vi "construct data interface.vi"(8 "error in":errorcluster, 10 "allocation specification":T1[](array[typedef])) -> (0 "error out":errorcluster, 3 "data table out":T3)   [LabVIEW 2013, in "tag bus.lvlib" / "data table.lvlib"]
doc: "Creates a data table based on the number of tags provided by the allocation specification."
uses:
  data table.lvlib
  data table.ctl
  allocation specification.ctl
  tag/Data Type.ctl
  tag/tag descriptor.lvclass
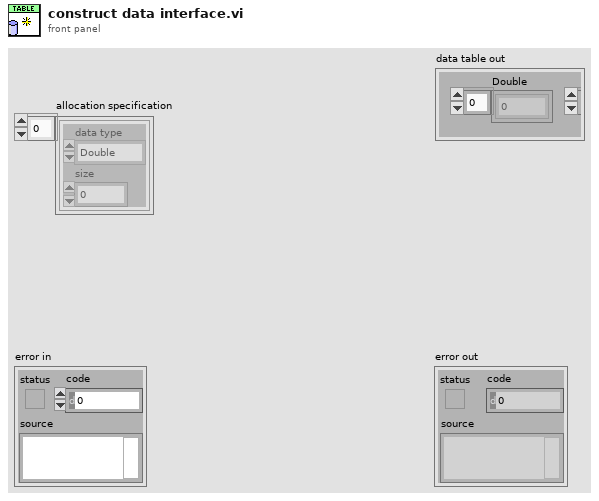
[diagram p1: front panel]
types:
  T1 = typedef "tag bus.lvlib/data table.lvlib/allocation specification.ctl" = cluster{"data type":T2, "size":i32}
  T2 = typedef "tag bus.lvlib/tag descriptor.lvclass/Data Type.ctl" = enum16{"Double", "Single", "I64", "I32", "I16", "I8", "U64", "U32", "U16", "U8", "Boolean", "String", "Array of Double", "Array of Single", "Array of I64", "Array of I32", "Array of I16", "Array of I8", "Array of U64", "Array of U32", "Array of U16", "Array of U8", "Array of Boolean", "Array of String"}
  T3 = typedef "tag bus.lvlib/data table.lvlib/data table.ctl" = cluster{"Double":dbl[], "Single":sgl[], "I64":i64[], "I32":i32[], "I16":i16[], "I8":i8[], "U64":u64[], "U32":u32[], "U16":u16[], "U8":u8[], "Boolean":bool[], "String":string[], "Array of Double":cluster{"DBL Array":dbl[]}[], "Array of Single":cluster{"SGL Array":sgl[]}[], "Array of I64":cluster{"I64 Array":i64[]}[], "Array of I32":cluster{"I32 Array":i32[]}[], "Array of I16":cluster{"I16 Array":i16[]}[], "Array of I8":cluster{"I8 Array":i8[]}[], "Array of U64":cluster{"U64 Array":u64[]}[], "Array of U32":cluster{"U32 Array":u32[]}[], "Array of U16":cluster{"U16 Array":u16[]}[], "Array of U8":cluster{"U8 Array":u8[]}[], "Array of Boolean":cluster{"Boolean Array":bool[]}[], "Array of String":cluster{"String Array":string[]}[]}
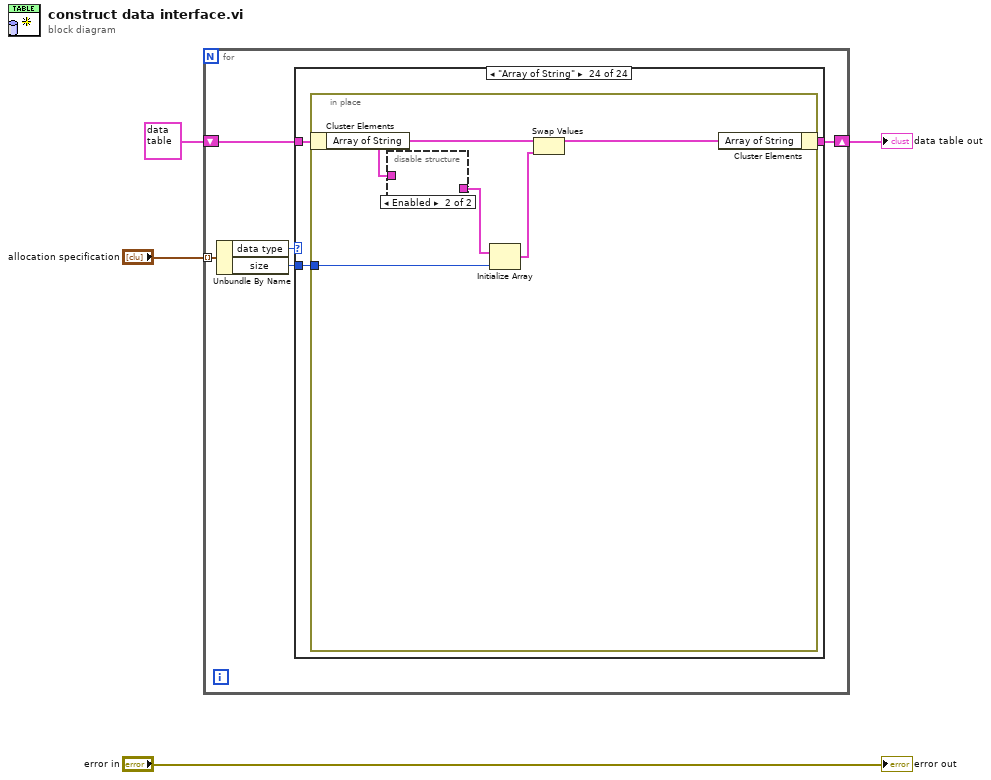
[diagram p0: block diagram]
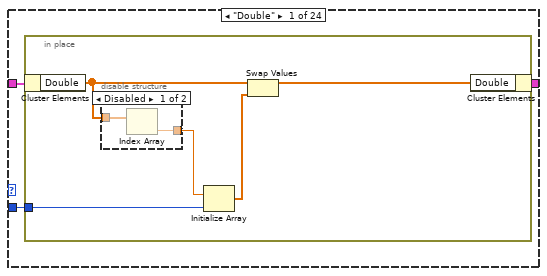
[diagram p2: hidden frame]
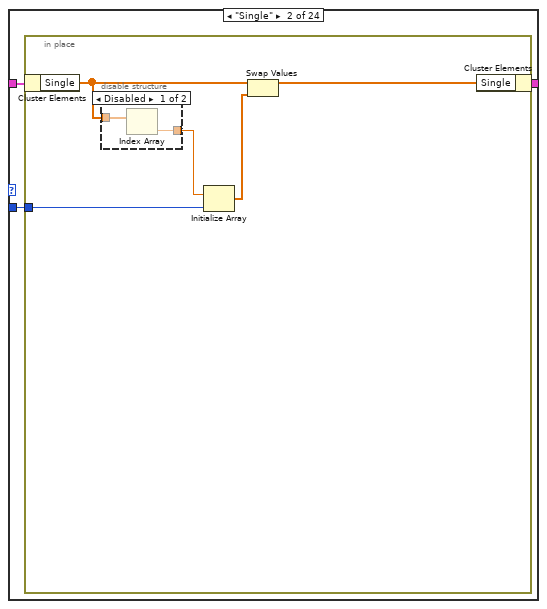
[diagram p4: hidden frame]
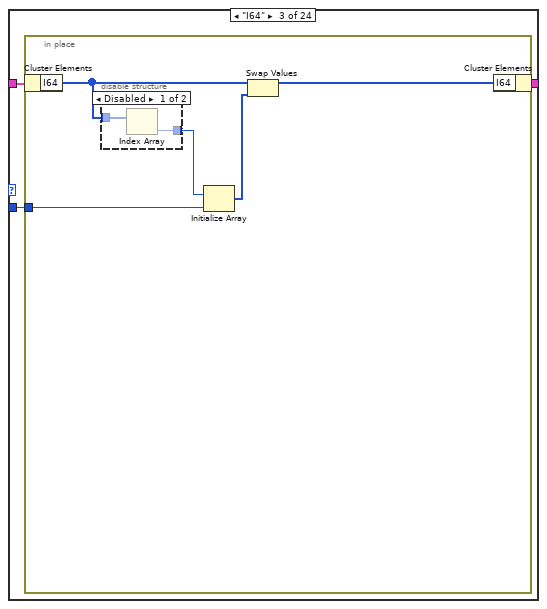
[diagram p6: hidden frame]
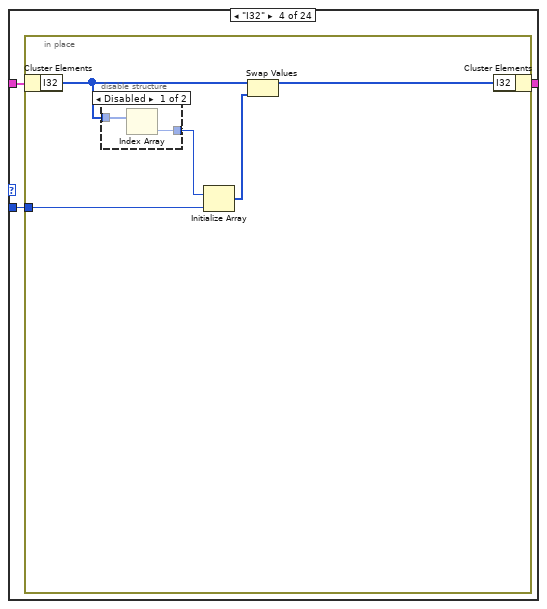
[diagram p8: hidden frame]
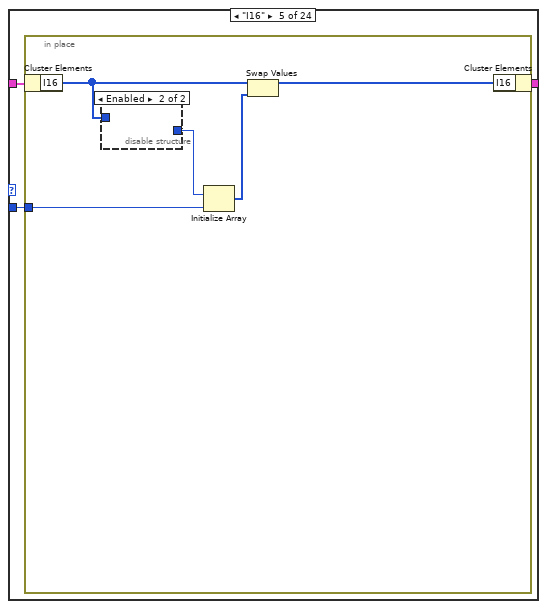
[diagram p10: hidden frame]
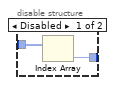
[diagram p11: hidden frame]
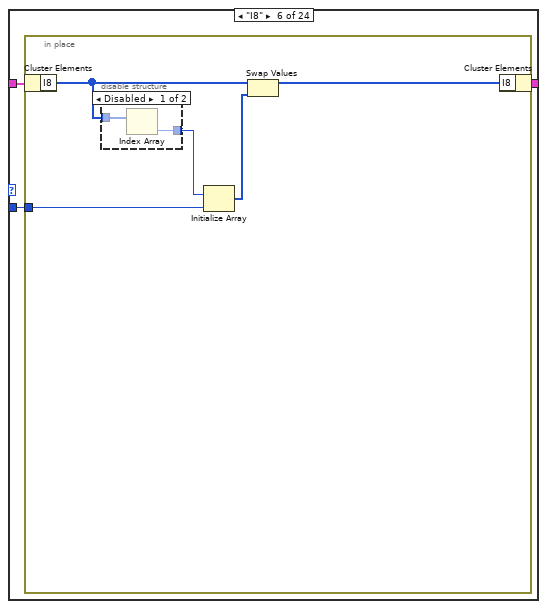
[diagram p12: hidden frame]
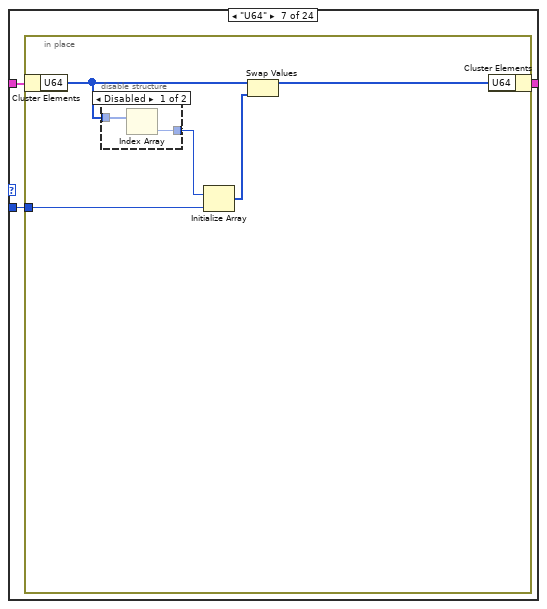
[diagram p14: hidden frame]
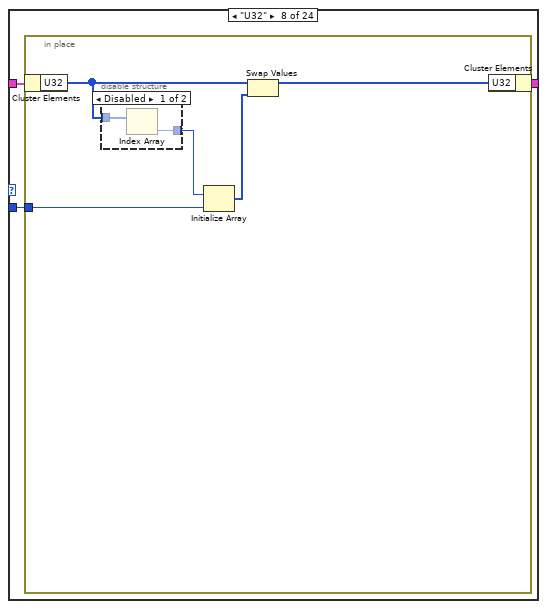
[diagram p16: hidden frame]
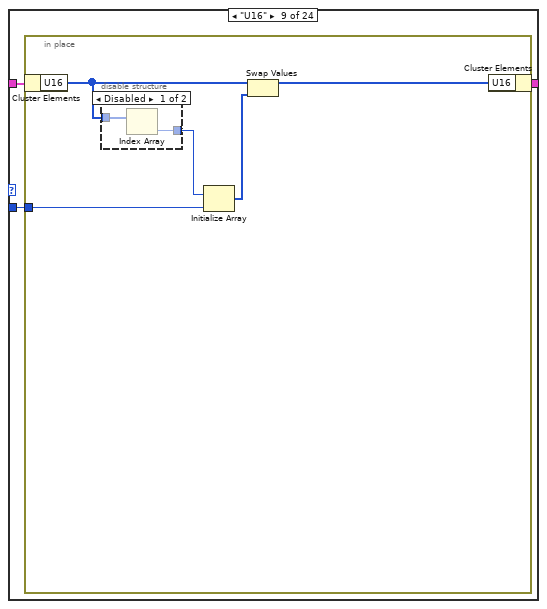
[diagram p18: hidden frame]
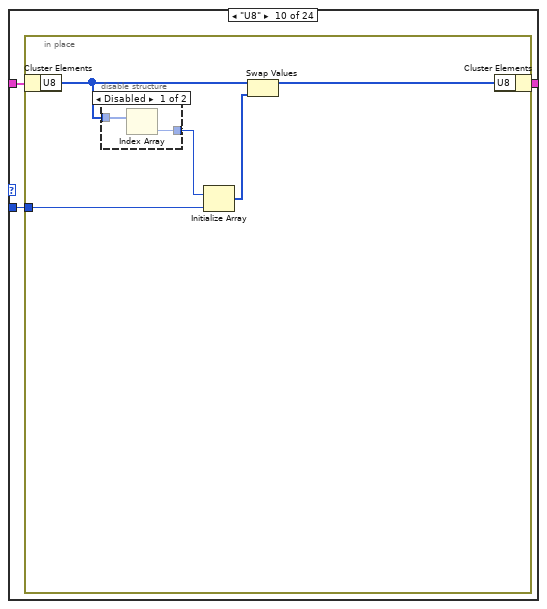
[diagram p20: hidden frame]
diagram:
  n1 = for {
    shift-right: [w6] -> w2
    shift-left: T3 {"Double"=[], "Single"=[], "I64"=[], "I32"=[], "I16"=[], "I8"=[], "U64"=[], "U32"=[], "U16"=[], "U8"=[], "Boolean"=[], "String"=[], "Array of Double"=[], "Array of Single"=[], "Array of I64"=[], "Array of I32"=[], "Array of I16"=[], "Array of I8"=[], "Array of U64"=[], "Array of U32"=[], "Array of U16"=[], "Array of U8"=[], "Array of Boolean"=[], "Array of String"=[]} ("Data Interface in") -> [w7]
    tunnel: "allocation specification" -> [w9] mode=indexing
    n2 = Unbundle By Name(w9) -> ("data type"=w8:T2, "size"=w5:i32)
    n3 = case shown="\"Array of String\"" w8 {
      tunnel: w7 -> [w11 w21 w31 w41 w51 w61 w71 w81 w91 w101 w111 w121 w131 w141 w151 w161 w171 w181 w191 w201 w211 w221 w231 w241]
      tunnel: [w12 w22 w32 w42 w52 w62 w72 w82 w92 w102 w112 w122 w132 w142 w152 w162 w172 w182 w192 w202 w212 w222 w232 w242] -> w6
      tunnel: w5 -> [w10 w20 w30 w40 w50 w60 w70 w80 w90 w100 w110 w120 w130 w140 w150 w160 w170 w180 w190 w200 w210 w220 w230 w240]
      frame "Double" {
        n4 = in-place {
          in-place-border: w10 -> [w17]
          n5 = in-place-cluster #1(w11) -> ("Double"=w15:dbl[])
          n6 = disable-structure shown="Disabled" {
            disable-tunnel: w15 -> [w19 _]
            disable-tunnel: [w18 _] -> w16
            frame Disabled {
              n7 = Index Array(array=w19) -> (element=w18:dbl)  [unwired: 1 in]
            }
            frame Enabled {
            }
          }
          n8 = Initialize Array(w16, w17) -> (w13:dbl[])
          n9 = Swap Values(12:w15, 14:w13) -> (1:w14:dbl[])  [unwired: 1 in, 1 out]
          n10 = in-place-cluster #1("Double"=w14) -> (w12:T3)
        }
      }
      frame "Single" {
        n11 = in-place {
          in-place-border: w20 -> [w27]
          n12 = in-place-cluster #2(w21) -> ("Single"=w25:sgl[])
          n13 = disable-structure shown="Disabled" {
            disable-tunnel: w25 -> [w29 _]
            disable-tunnel: [w28 _] -> w26
            frame Disabled {
              n14 = Index Array(array=w29) -> (element=w28:sgl)  [unwired: 1 in]
            }
            frame Enabled {
            }
          }
          n15 = Initialize Array(w26, w27) -> (w23:sgl[])
          n16 = Swap Values(12:w25, 14:w23) -> (1:w24:sgl[])  [unwired: 1 in, 1 out]
          n17 = in-place-cluster #2("Single"=w24) -> (w22:T3)
        }
      }
      frame "I64" {
        n18 = in-place {
          in-place-border: w30 -> [w37]
          n19 = in-place-cluster #3(w31) -> ("I64"=w35:i64[])
          n20 = disable-structure shown="Disabled" {
            disable-tunnel: w35 -> [w39 _]
            disable-tunnel: [w38 _] -> w36
            frame Disabled {
              n21 = Index Array(array=w39) -> (element=w38:i64)  [unwired: 1 in]
            }
            frame Enabled {
            }
          }
          n22 = Initialize Array(w36, w37) -> (w33:i64[])
          n23 = Swap Values(12:w35, 14:w33) -> (1:w34:i64[])  [unwired: 1 in, 1 out]
          n24 = in-place-cluster #3("I64"=w34) -> (w32:T3)
        }
      }
      frame "I32" {
        n25 = in-place {
          in-place-border: w40 -> [w47]
          n26 = in-place-cluster #4(w41) -> ("I32"=w45:i32[])
          n27 = disable-structure shown="Disabled" {
            disable-tunnel: w45 -> [w49 _]
            disable-tunnel: [w48 _] -> w46
            frame Disabled {
              n28 = Index Array(array=w49) -> (element=w48:i32)  [unwired: 1 in]
            }
            frame Enabled {
            }
          }
          n29 = Initialize Array(w46, w47) -> (w43:i32[])
          n30 = Swap Values(12:w45, 14:w43) -> (1:w44:i32[])  [unwired: 1 in, 1 out]
          n31 = in-place-cluster #4("I32"=w44) -> (w42:T3)
        }
      }
      frame "I16" {
        n32 = in-place {
          in-place-border: w50 -> [w57]
          n33 = in-place-cluster #5(w51) -> ("I16"=w55:i16[])
          n34 = disable-structure shown="Enabled" {
            disable-tunnel: w55 -> [w59 _]
            disable-tunnel: [w58 _] -> w56
            frame Disabled {
              n35 = Index Array(array=w59) -> (element=w58:i16)  [unwired: 1 in]
            }
            frame Enabled {
            }
          }
          n36 = Initialize Array(w56, w57) -> (w53:i16[])
          n37 = Swap Values(12:w55, 14:w53) -> (1:w54:i16[])  [unwired: 1 in, 1 out]
          n38 = in-place-cluster #5("I16"=w54) -> (w52:T3)
        }
      }
      frame "I8" {
        n39 = in-place {
          in-place-border: w60 -> [w67]
          n40 = in-place-cluster #6(w61) -> ("I8"=w65:i8[])
          n41 = disable-structure shown="Disabled" {
            disable-tunnel: w65 -> [w69 _]
            disable-tunnel: [w68 _] -> w66
            frame Disabled {
              n42 = Index Array(array=w69) -> (element=w68:i8)  [unwired: 1 in]
            }
            frame Enabled {
            }
          }
          n43 = Initialize Array(w66, w67) -> (w63:i8[])
          n44 = Swap Values(12:w65, 14:w63) -> (1:w64:i8[])  [unwired: 1 in, 1 out]
          n45 = in-place-cluster #6("I8"=w64) -> (w62:T3)
        }
      }
      frame "U64" {
        n46 = in-place {
          in-place-border: w70 -> [w77]
          n47 = in-place-cluster #7(w71) -> ("U64"=w75:u64[])
          n48 = disable-structure shown="Disabled" {
            disable-tunnel: w75 -> [w79 _]
            disable-tunnel: [w78 _] -> w76
            frame Disabled {
              n49 = Index Array(array=w79) -> (element=w78:u64)  [unwired: 1 in]
            }
            frame Enabled {
            }
          }
          n50 = Initialize Array(w76, w77) -> (w73:u64[])
          n51 = Swap Values(12:w75, 14:w73) -> (1:w74:u64[])  [unwired: 1 in, 1 out]
          n52 = in-place-cluster #7("U64"=w74) -> (w72:T3)
        }
      }
      frame "U32" {
        n53 = in-place {
          in-place-border: w80 -> [w87]
          n54 = in-place-cluster #8(w81) -> ("U32"=w85:u32[])
          n55 = disable-structure shown="Disabled" {
            disable-tunnel: w85 -> [w89 _]
            disable-tunnel: [w88 _] -> w86
            frame Disabled {
              n56 = Index Array(array=w89) -> (element=w88:u32)  [unwired: 1 in]
            }
            frame Enabled {
            }
          }
          n57 = Initialize Array(w86, w87) -> (w83:u32[])
          n58 = Swap Values(12:w85, 14:w83) -> (1:w84:u32[])  [unwired: 1 in, 1 out]
          n59 = in-place-cluster #8("U32"=w84) -> (w82:T3)
        }
      }
      frame "U16" {
        n60 = in-place {
          in-place-border: w90 -> [w97]
          n61 = in-place-cluster #9(w91) -> ("U16"=w95:u16[])
          n62 = disable-structure shown="Disabled" {
            disable-tunnel: w95 -> [w99 _]
            disable-tunnel: [w98 _] -> w96
            frame Disabled {
              n63 = Index Array(array=w99) -> (element=w98:u16)  [unwired: 1 in]
            }
            frame Enabled {
            }
          }
          n64 = Initialize Array(w96, w97) -> (w93:u16[])
          n65 = Swap Values(12:w95, 14:w93) -> (1:w94:u16[])  [unwired: 1 in, 1 out]
          n66 = in-place-cluster #9("U16"=w94) -> (w92:T3)
        }
      }
      frame "U8" {
        n67 = in-place {
          in-place-border: w100 -> [w107]
          n68 = in-place-cluster #10(w101) -> ("U8"=w105:u8[])
          n69 = disable-structure shown="Disabled" {
            disable-tunnel: w105 -> [w109 _]
            disable-tunnel: [w108 _] -> w106
            frame Disabled {
              n70 = Index Array(array=w109) -> (element=w108:u8)  [unwired: 1 in]
            }
            frame Enabled {
            }
          }
          n71 = Initialize Array(w106, w107) -> (w103:u8[])
          n72 = Swap Values(12:w105, 14:w103) -> (1:w104:u8[])  [unwired: 1 in, 1 out]
          n73 = in-place-cluster #10("U8"=w104) -> (w102:T3)
        }
      }
      frame "String" {
        n74 = in-place {
          in-place-border: w110 -> [w117]
          n75 = in-place-cluster #11(w111) -> ("String"=w115:string[])
          n76 = disable-structure shown="Disabled" {
            disable-tunnel: w115 -> [w119 _]
            disable-tunnel: [w118 _] -> w116
            frame Disabled {
              n77 = Index Array(array=w119) -> (element=w118:string)  [unwired: 1 in]
            }
            frame Enabled {
            }
          }
          n78 = Initialize Array(w116, w117) -> (w113:string[])
          n79 = Swap Values(12:w115, 14:w113) -> (1:w114:string[])  [unwired: 1 in, 1 out]
          n80 = in-place-cluster #11("String"=w114) -> (w112:T3)
        }
      }
      frame "Boolean" {
        n81 = in-place {
          in-place-border: w120 -> [w127]
          n82 = in-place-cluster #12(w121) -> ("Boolean"=w125:bool[])
          n83 = disable-structure shown="Disabled" {
            disable-tunnel: w125 -> [w129 _]
            disable-tunnel: [w128 _] -> w126
            frame Disabled {
              n84 = Index Array(array=w129) -> (element=w128:bool)  [unwired: 1 in]
            }
            frame Enabled {
            }
          }
          n85 = Initialize Array(w126, w127) -> (w123:bool[])
          n86 = Swap Values(12:w125, 14:w123) -> (1:w124:bool[])  [unwired: 1 in, 1 out]
          n87 = in-place-cluster #12("Boolean"=w124) -> (w122:T3)
        }
      }
      frame "Array of U8" {
        n88 = in-place {
          in-place-border: w130 -> [w137]
          n89 = in-place-cluster #13(w131) -> ("Array of U8"=w135:cluster{"U8 Array":u8[]}[])
          n90 = disable-structure shown="Disabled" {
            disable-tunnel: w135 -> [w139 _]
            disable-tunnel: [w138 _] -> w136
            frame Disabled {
              n91 = Index Array(array=w139) -> (element=w138:cluster{"U8 Array":u8[]})  [unwired: 1 in]
            }
            frame Enabled {
            }
          }
          n92 = Initialize Array(w136, w137) -> (w133:cluster{"U8 Array":u8[]}[])
          n93 = Swap Values(12:w135, 14:w133) -> (1:w134:cluster{"U8 Array":u8[]}[])  [unwired: 1 in, 1 out]
          n94 = in-place-cluster #13("Array of U8"=w134) -> (w132:T3)
        }
      }
      frame "Array of U16" {
        n95 = in-place {
          in-place-border: w140 -> [w147]
          n96 = in-place-cluster #14(w141) -> ("Array of U16"=w145:cluster{"U16 Array":u16[]}[])
          n97 = disable-structure shown="Disabled" {
            disable-tunnel: w145 -> [w149 _]
            disable-tunnel: [w148 _] -> w146
            frame Disabled {
              n98 = Index Array(array=w149) -> (element=w148:cluster{"U16 Array":u16[]})  [unwired: 1 in]
            }
            frame Enabled {
            }
          }
          n99 = Initialize Array(w146, w147) -> (w143:cluster{"U16 Array":u16[]}[])
          n100 = Swap Values(12:w145, 14:w143) -> (1:w144:cluster{"U16 Array":u16[]}[])  [unwired: 1 in, 1 out]
          n101 = in-place-cluster #14("Array of U16"=w144) -> (w142:T3)
        }
      }
      frame "Array of U32" {
        n102 = in-place {
          in-place-border: w150 -> [w157]
          n103 = in-place-cluster #15(w151) -> ("Array of U32"=w155:cluster{"U32 Array":u32[]}[])
          n104 = disable-structure shown="Disabled" {
            disable-tunnel: w155 -> [w159 _]
            disable-tunnel: [w158 _] -> w156
            frame Disabled {
              n105 = Index Array(array=w159) -> (element=w158:cluster{"U32 Array":u32[]})  [unwired: 1 in]
            }
            frame Enabled {
            }
          }
          n106 = Initialize Array(w156, w157) -> (w153:cluster{"U32 Array":u32[]}[])
          n107 = Swap Values(12:w155, 14:w153) -> (1:w154:cluster{"U32 Array":u32[]}[])  [unwired: 1 in, 1 out]
          n108 = in-place-cluster #15("Array of U32"=w154) -> (w152:T3)
        }
      }
      frame "Array of U64" {
        n109 = in-place {
          in-place-border: w160 -> [w167]
          n110 = in-place-cluster #16(w161) -> ("Array of U64"=w165:cluster{"U64 Array":u64[]}[])
          n111 = disable-structure shown="Disabled" {
            disable-tunnel: w165 -> [w169 _]
            disable-tunnel: [w168 _] -> w166
            frame Disabled {
              n112 = Index Array(array=w169) -> (element=w168:cluster{"U64 Array":u64[]})  [unwired: 1 in]
            }
            frame Enabled {
            }
          }
          n113 = Initialize Array(w166, w167) -> (w163:cluster{"U64 Array":u64[]}[])
          n114 = Swap Values(12:w165, 14:w163) -> (1:w164:cluster{"U64 Array":u64[]}[])  [unwired: 1 in, 1 out]
          n115 = in-place-cluster #16("Array of U64"=w164) -> (w162:T3)
        }
      }
      frame "Array of I64" {
        n116 = in-place {
          in-place-border: w170 -> [w177]
          n117 = in-place-cluster #17(w171) -> ("Array of I64"=w175:cluster{"I64 Array":i64[]}[])
          n118 = disable-structure shown="Disabled" {
            disable-tunnel: w175 -> [w179 _]
            disable-tunnel: [w178 _] -> w176
            frame Disabled {
              n119 = Index Array(array=w179) -> (element=w178:cluster{"I64 Array":i64[]})  [unwired: 1 in]
            }
            frame Enabled {
            }
          }
          n120 = Initialize Array(w176, w177) -> (w173:cluster{"I64 Array":i64[]}[])
          n121 = Swap Values(12:w175, 14:w173) -> (1:w174:cluster{"I64 Array":i64[]}[])  [unwired: 1 in, 1 out]
          n122 = in-place-cluster #17("Array of I64"=w174) -> (w172:T3)
        }
      }
      frame "Array of I32" {
        n123 = in-place {
          in-place-border: w180 -> [w187]
          n124 = in-place-cluster #18(w181) -> ("Array of I32"=w185:cluster{"I32 Array":i32[]}[])
          n125 = disable-structure shown="Disabled" {
            disable-tunnel: w185 -> [w189 _]
            disable-tunnel: [w188 _] -> w186
            frame Disabled {
              n126 = Index Array(array=w189) -> (element=w188:cluster{"I32 Array":i32[]})  [unwired: 1 in]
            }
            frame Enabled {
            }
          }
          n127 = Initialize Array(w186, w187) -> (w183:cluster{"I32 Array":i32[]}[])
          n128 = Swap Values(12:w185, 14:w183) -> (1:w184:cluster{"I32 Array":i32[]}[])  [unwired: 1 in, 1 out]
          n129 = in-place-cluster #18("Array of I32"=w184) -> (w182:T3)
        }
      }
      frame "Array of I16" {
        n130 = in-place {
          in-place-border: w190 -> [w197]
          n131 = in-place-cluster #19(w191) -> ("Array of I16"=w195:cluster{"I16 Array":i16[]}[])
          n132 = disable-structure shown="Disabled" {
            disable-tunnel: w195 -> [w199 _]
            disable-tunnel: [w198 _] -> w196
            frame Disabled {
              n133 = Index Array(array=w199) -> (element=w198:cluster{"I16 Array":i16[]})  [unwired: 1 in]
            }
            frame Enabled {
            }
          }
          n134 = Initialize Array(w196, w197) -> (w193:cluster{"I16 Array":i16[]}[])
          n135 = Swap Values(12:w195, 14:w193) -> (1:w194:cluster{"I16 Array":i16[]}[])  [unwired: 1 in, 1 out]
          n136 = in-place-cluster #19("Array of I16"=w194) -> (w192:T3)
        }
      }
      frame "Array of I8" {
        n137 = in-place {
          in-place-border: w200 -> [w207]
          n138 = in-place-cluster #20(w201) -> ("Array of I8"=w205:cluster{"I8 Array":i8[]}[])
          n139 = disable-structure shown="Disabled" {
            disable-tunnel: w205 -> [w209 _]
            disable-tunnel: [w208 _] -> w206
            frame Disabled {
              n140 = Index Array(array=w209) -> (element=w208:cluster{"I8 Array":i8[]})  [unwired: 1 in]
            }
            frame Enabled {
            }
          }
          n141 = Initialize Array(w206, w207) -> (w203:cluster{"I8 Array":i8[]}[])
          n142 = Swap Values(12:w205, 14:w203) -> (1:w204:cluster{"I8 Array":i8[]}[])  [unwired: 1 in, 1 out]
          n143 = in-place-cluster #20("Array of I8"=w204) -> (w202:T3)
        }
      }
      frame "Array of Double" {
        n144 = in-place {
          in-place-border: w210 -> [w217]
          n145 = in-place-cluster #21(w211) -> ("Array of Double"=w215:cluster{"DBL Array":dbl[]}[])
          n146 = disable-structure shown="Disabled" {
            disable-tunnel: w215 -> [w219 _]
            disable-tunnel: [w218 _] -> w216
            frame Disabled {
              n147 = Index Array(array=w219) -> (element=w218:cluster{"DBL Array":dbl[]})  [unwired: 1 in]
            }
            frame Enabled {
            }
          }
          n148 = Initialize Array(w216, w217) -> (w213:cluster{"DBL Array":dbl[]}[])
          n149 = Swap Values(12:w215, 14:w213) -> (1:w214:cluster{"DBL Array":dbl[]}[])  [unwired: 1 in, 1 out]
          n150 = in-place-cluster #21("Array of Double"=w214) -> (w212:T3)
        }
      }
      frame "Array of Single" {
        n151 = in-place {
          in-place-border: w220 -> [w227]
          n152 = in-place-cluster #22(w221) -> ("Array of Single"=w225:cluster{"SGL Array":sgl[]}[])
          n153 = disable-structure shown="Disabled" {
            disable-tunnel: w225 -> [w229 _]
            disable-tunnel: [w228 _] -> w226
            frame Disabled {
              n154 = Index Array(array=w229) -> (element=w228:cluster{"SGL Array":sgl[]})  [unwired: 1 in]
            }
            frame Enabled {
            }
          }
          n155 = Initialize Array(w226, w227) -> (w223:cluster{"SGL Array":sgl[]}[])
          n156 = Swap Values(12:w225, 14:w223) -> (1:w224:cluster{"SGL Array":sgl[]}[])  [unwired: 1 in, 1 out]
          n157 = in-place-cluster #22("Array of Single"=w224) -> (w222:T3)
        }
      }
      frame "Array of Boolean" {
        n158 = in-place {
          in-place-border: w230 -> [w237]
          n159 = in-place-cluster #23(w231) -> ("Array of Boolean"=w235:cluster{"Boolean Array":bool[]}[])
          n160 = disable-structure shown="Disabled" {
            disable-tunnel: w235 -> [w239 _]
            disable-tunnel: [w238 _] -> w236
            frame Disabled {
              n161 = Index Array(array=w239) -> (element=w238:cluster{"Boolean Array":bool[]})  [unwired: 1 in]
            }
            frame Enabled {
            }
          }
          n162 = Initialize Array(w236, w237) -> (w233:cluster{"Boolean Array":bool[]}[])
          n163 = Swap Values(12:w235, 14:w233) -> (1:w234:cluster{"Boolean Array":bool[]}[])  [unwired: 1 in, 1 out]
          n164 = in-place-cluster #23("Array of Boolean"=w234) -> (w232:T3)
        }
      }
      frame "Array of String" {
        n165 = in-place {
          in-place-border: w240 -> [w247]
          n166 = in-place-cluster #24(w241) -> ("Array of String"=w245:cluster{"String Array":string[]}[])
          n167 = disable-structure shown="Enabled" {
            disable-tunnel: w245 -> [w249 _]
            disable-tunnel: [w248 _] -> w246
            frame Disabled {
              n168 = Index Array(array=w249) -> (element=w248:cluster{"String Array":string[]})  [unwired: 1 in]
            }
            frame Enabled {
            }
          }
          n169 = Initialize Array(w246, w247) -> (w243:cluster{"String Array":string[]}[])
          n170 = Swap Values(12:w245, 14:w243) -> (1:w244:cluster{"String Array":string[]}[])  [unwired: 1 in, 1 out]
          n171 = in-place-cluster #24("Array of String"=w244) -> (w242:T3)
        }
      }
    }
  }
  "data table out" <- w2
  "error out" <- "error in"
